vi "Receive.vi"(7 "Device Address":u8, 8 "error in (no error)":errorcluster, 9 "I2Cflags":T1 caption="I2C Flags" items=["None"=0, "START"=2, "REPEATED START"=3, "STOP"=4, "START AND STOP"=6], 10 "Bytes To Read":u32, 11 "I2COUSBSim in":refnum<class "I2COUSBSim.lvclass">) -> (0 "error out":errorcluster, 1 "Status":string, 2 "Buffer":u8[](array[numeric]), 3 "I2COUSBSim out":refnum<class "I2COUSBSim.lvclass">, 5 "Byte Returned":u32)   [LabVIEW 2020, in "I2COUSB.lvlib" / "I2COUSBSim.lvclass"]
doc: "Receive Data"
uses:
  I2COUSBSim.lvclass
  II2COUSB/II2COUSB/I2CFlags.ctl
  I2COUSBSim.lvclass/I2COUSBSim.ctl
  II2COUSB/II2COUSB/II2COUSB.lvclass
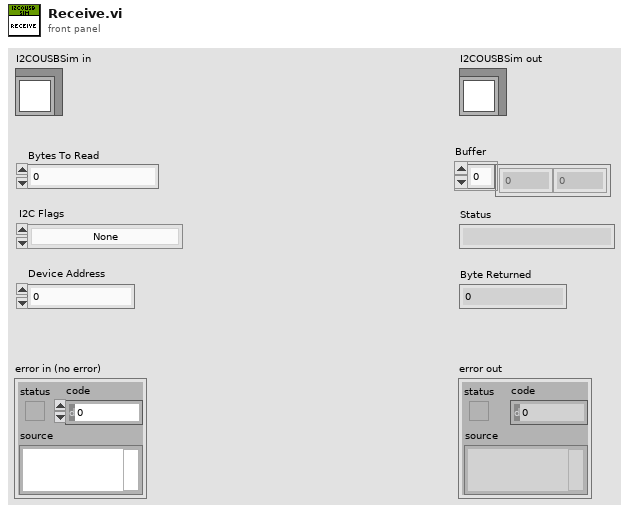
[diagram p1: front panel]
types:
  T1 = typedef "II2COUSB.lvlib/II2COUSB.lvclass/I2CFlags.ctl" = u8
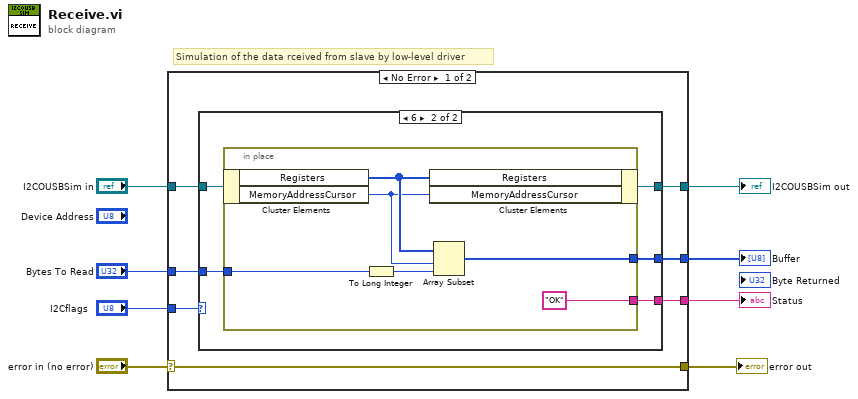
[diagram p0: block diagram]
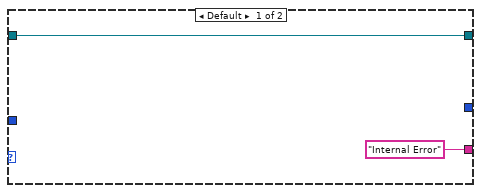
[diagram p2: hidden frame]
diagram:
  # "Simulation of the data rceived from slave by low-level driver"
  n1 = case shown="No Error" "error in (no error)" {
    selector: "error in (no error)" -> [w9 w29]
    tunnel: "I2COUSBSim in" -> [w13 w30]
    tunnel: [w14 w30] -> w7
    tunnel: [w9 w29] -> w5
    tunnel: "I2Cflags" -> [w15 _]
    tunnel: "Bytes To Read" -> [w12 _]
    tunnel: [w11 _] -> w2
    tunnel: [w10 _] -> w1
    frame No Error {
      n2 = case shown="6" w15 {
        tunnel: [w17 w19] -> w14
        tunnel: w13 -> [w17 w22]
        tunnel: w12 -> [_ w21]
        tunnel: [_ w20] -> w11
        tunnel: ["Internal Error" w18] -> w10
        frame Default {
        }
        frame 6 {
          n3 = in-place {
            in-place-border: w21 -> [w26]
            in-place-border: [w24] -> w20
            in-place-border: ["OK"] -> w18
            n4 = in-place-cluster #1(w22) -> ("Registers"=w28:u8[], "MemoryAddressCursor"=w27:i32)
            n5 = To Long Integer(number=w26) -> (32bit integer=w25:i32)
            n6 = in-place-cluster #1("Registers"=w28, "MemoryAddressCursor"=w27) -> (w19:refnum<class "I2COUSBSim.lvclass">)
            n7 = Array Subset(array=w28, index=w27, length=w25) -> (w24:u8[])
          }
        }
      }
    }
    frame Error {
    }
  }
  "error out" <- w5
  "I2COUSBSim out" <- w7
  "Buffer" <- w2
  "Status" <- w1
